vi "SimpleOscillate.vi"() -> ()   [LabVIEW 2010]
uses:
  Motion/EnableSingle.vi
panel:
  in  "axis name":string="X"
  in  "Disconnect After?":bool
  in  "Execute In Back-\nground Thread":bool
  in  "NumFreqs":i32=2
  in  "Cycles":i32=2
  in  "Distance":dbl=50.0
  in  "Frequency":dbl=1.0
  out "error out":errorcluster
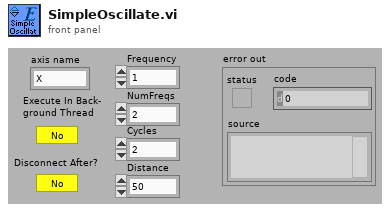
[diagram p1: front panel]
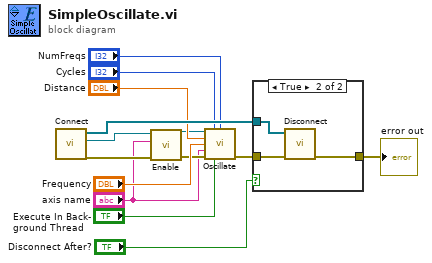
[diagram p0: block diagram]
diagram:
  n1 = call "Connect.vi"() -> ("error out"=w3:errorcluster, "controller"=w2:refnum<k24>, "controllers"=w14:refnum<k24>[])  [unwired: 9 in]
  n2 = call-poly "Enable.vi"("error in (no error)"=w3, "axis name"="axis name", "controller in"=w2) -> ("error out"=w5:errorcluster, "controller out"=w4:refnum<k24>)  [unwired: 7 in]
  n3 = call "Oscillate.vi"("controller in"=w4, "Cycles"="Cycles", "NumFreqs"="NumFreqs", "Distance"="Distance", "Frequency"="Frequency", "axis name"="axis name", "error in (no error)"=w5, "executeInBgThread"="Execute In Back-\nground Thread") -> ("error out"=w12:errorcluster)  [unwired: 6 in, 1 out]
  n4 = case shown="True" "Disconnect After?" {
    tunnel: w14 -> [_ w18]
    tunnel: [w15 w17] -> w13
    tunnel: w12 -> [w15 w16]
    frame False {
    }
    frame True {
      n5 = call "Disconnect.vi"("error in (no error)"=w16, "controllers"=w18) -> ("error out"=w17:errorcluster)  [unwired: 9 in]
    }
  }
  "error out" <- w13
